vi "Clear Specific Error.vi"(1 "Error Numbers Array (emtpy)":i32[](array[numeric]), 2 "Specific Error Number (0: none)":i32, 7 "error in":errorcluster, 12 "EnableMsgPopup":bool caption="Msg Popup? (f)", 13 "Message":string) -> (6 "Error Cleared?":bool, 8 "error out":errorcluster)   [LabVIEW 2011]
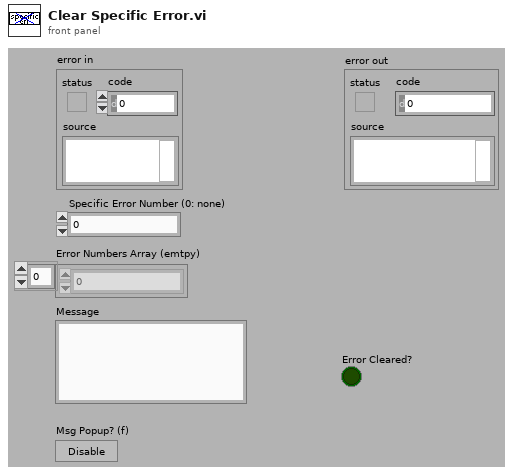
[diagram p1: front panel]
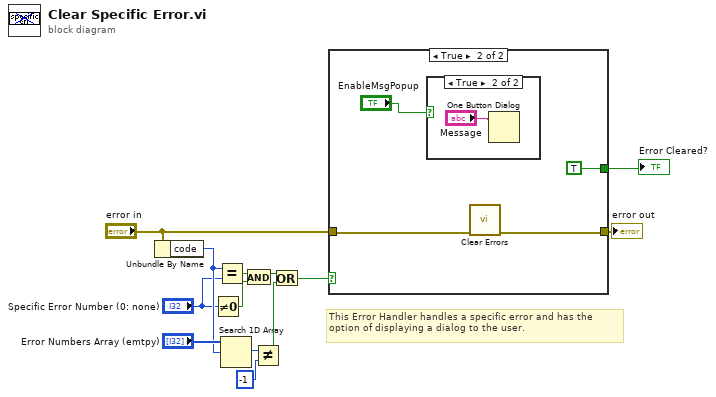
[diagram p0: block diagram]
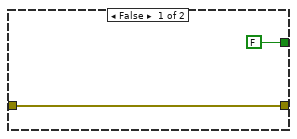
[diagram p2: hidden frame]
diagram:
  # "This Error Handler handles a specific error and has the option of displaying a dialog to the user."
  n1 = Unbundle By Name("error in") -> ("code"=w8:i32)
  n2 = Not Equal To 0?(x="Specific Error Number (0: none)") -> (x != 0?=w2:bool)
  n3 = Equal?(x=w8, y="Specific Error Number (0: none)") -> (x = y?=w10:bool)
  n4 = Search 1D Array(1D array="Error Numbers Array (emtpy)", element=w8) -> (index of element=w6:i32)  [unwired: 1 out]
  n5 = And(x=w10, y=w2) -> (x .and. y?=w3:bool)
  n6 = Not Equal?(x=w6, y=-1) -> (x != y?=w5:bool)
  n7 = Or(x=w3, y=w5) -> (x .or. y?=w4:bool)
  n8 = case shown="True" w4 {
    tunnel: "error in" -> [w15 w19]
    tunnel: [w15 w18] -> w12
    tunnel: [FALSE ("true") TRUE ("true")] -> w11
    frame False {
    }
    frame True {
      n9 = case shown="True" "EnableMsgPopup" {
        frame False {
        }
        frame True {
          n10 = One Button Dialog(message="Message") -> ()  [unwired: 2 out]
        }
      }
      n11 = call <vilib>:"Clear Errors.vi"("error in (no error)"=w19) -> ("error out"=w18:errorcluster)  [unwired: 6 out]
    }
  }
  "error out" <- w12
  "Error Cleared?" <- w11
